vi "Save Image.vi"(8 "error in (no error)":errorcluster, 11 "IMAQ Display in":refnum<class "POLARIS TA Focus Display.lvclass">) -> (0 "error out":errorcluster, 3 "IMAQ Display out":refnum<class "POLARIS TA Focus Display.lvclass">)   [LabVIEW 2014, in "POLARIS TA Focus Display.lvlib" / "POLARIS TA Focus Display.lvclass"]
uses:
  POLARIS TA Focus Display.lvclass
  POLARIS TA Focus Display.lvclass/POLARIS TA Focus Display.ctl
  Display Actors/HIJ Vision Display/HIJ Vision Display/HIJ Vision Display.lvclass/HIJ Vision Display.ctl
  Display Actors/HIJ Vision Display/HIJ Vision Display/Write Image Name Prefix.vi
  Read Results in Filename.vi
  Display Actors/HIJ IMAQdx Display/AF IMAQ Display/HIJ IMAQdx Display.lvclass
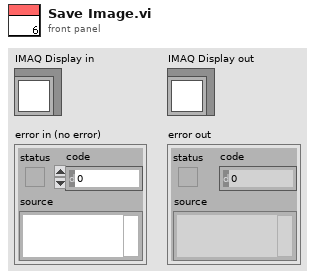
[diagram p1: front panel]
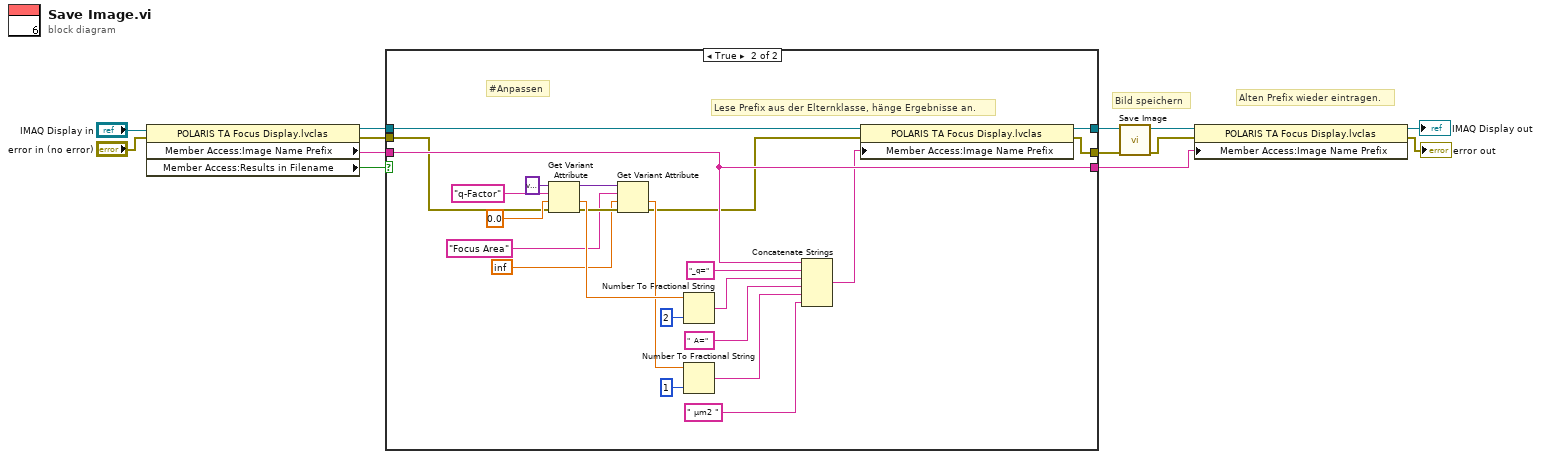
[diagram p0: block diagram]
diagram:
  # "Alten Prefix wieder eintragen."
  # "Bild speichern"
  n1 = property class="POLARIS TA Focus Display.lvclas"(reference="IMAQ Display in", error in="error in (no error)") -> (reference out=w10:refnum<class "POLARIS TA Focus Display.lvclass">, error out=w3:errorcluster, "Member Access:Image Name Prefix"=w13:string, "Member Access:Results in Filename"=w2:bool)
  n2 = case shown="True" w2 {
    tunnel: w13 -> [w14 w39]
    tunnel: w10 -> [w16 w37]
    tunnel: [w16 w22] -> w9
    tunnel: [w15 w20] -> w6
    tunnel: w3 -> [w15 w19]
    tunnel: [w14 w39] -> w1
    frame False {
    }
    frame True {
      # "#Anpassen"
      # "Lese Prefix aus der Elternklasse, hänge Ergebnisse an."
      n3 = Get Variant Attribute(Variant=variant ("variant"), name="q-Factor", default value (empty Variant)=0.0, error in=w19) -> (duplicate Variant=w26:variant, value=w38:dbl, error out=w28:errorcluster)  [unwired: 1 out]
      n4 = Get Variant Attribute(Variant=w26, name="Focus Area", default value (empty Variant)=inf, error in=w28) -> (value=w23:dbl, error out=w18:errorcluster)  [unwired: 2 out]
      n5 = Number To Fractional String(number=w38, precision (6)=i16 2 ("Genauigkeit (6)")) -> (F-format string=w35:string)  [unwired: 2 in]
      n6 = Number To Fractional String(number=w23, precision (6)=i16 1 ("Genauigkeit (6)")) -> (F-format string=w31:string)  [unwired: 2 in]
      n7 = Concatenate Strings(w39, "_q=" ("String"), w35, "  A=" ("String"), w31, " µm2 " ("String")) -> (w21:string)
      n8 = property class="POLARIS TA Focus Display.lvclas"(reference=w37, error in=w18, "Member Access:Image Name Prefix"=w21) -> (reference out=w22:refnum<class "POLARIS TA Focus Display.lvclass">, error out=w20:errorcluster)
    }
  }
  n9 = call-parent "Save Image.vi"("error in (no error)"=w6, "IMAQ Display in"=w9) -> ("error out"=w5:errorcluster, "IMAQ Display out"=w12:refnum<class "POLARIS TA Focus Display.lvclass">)  [unwired: 8 in]
  n10 = property class="POLARIS TA Focus Display.lvclas"(reference=w12, error in=w5, "Member Access:Image Name Prefix"=w1) -> (reference out=→"IMAQ Display out":refnum<class "POLARIS TA Focus Display.lvclass">, error out=→"error out":errorcluster)
